vi "Close.vi"(0 "reference in":refnum<class "GUI.lvclass">, 5 "error in (no error)":errorcluster) -> (14 "reference out":refnum<class "GUI.lvclass">, 15 "dt":u32, 19 "error out":errorcluster)   [LabVIEW 2019, in "GUI.lvclass"]
doc: "Destructor."
uses:
  GUI.lvclass
  GUI.lvclass/GUI.ctl
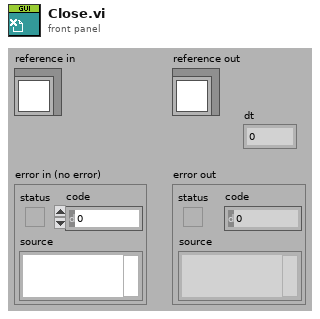
[diagram p1: front panel]
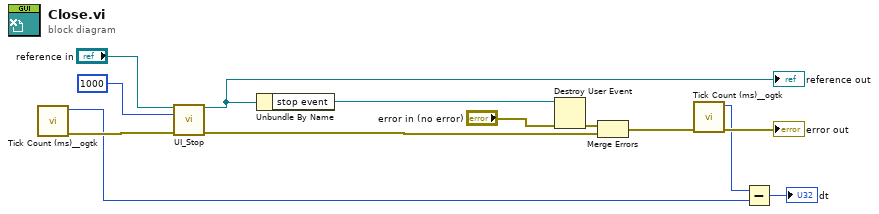
[diagram p0: block diagram]
diagram:
  n1 = call "Tick Count (ms)__ogtk.vi"() -> ("error out"=w6:errorcluster, "millisecond timer value"=w2:u32)  [unwired: 10 in]
  n2 = call "UI_Stop.vi"("reference in"="reference in", "timeout ms"=1000, "error in (no error)"=w6) -> ("reference out"=w9:refnum<class "GUI.lvclass">, "error out"=w8:errorcluster)  [unwired: 9 in, 2 out]
  "reference out" <- w9
  n3 = Unbundle By Name(w9) -> ("stop event"=w13:refnum<user-event>)
  n4 = Destroy User Event(user event=w13, error in="error in (no error)") -> (error out=w11:errorcluster)
  n5 = Merge Errors(w11, w8) -> (w5:errorcluster)
  n6 = call "Tick Count (ms)__ogtk.vi"("error in (no error)"=w5) -> ("error out"=→"error out":errorcluster, "millisecond timer value"=w3:u32)  [unwired: 9 in]
  n7 = Subtract(x=w3, y=w2) -> (x-y=→"dt":u32)
